vi "printgraph_V0.01.vi"(4 "AFR":refnum<vi>, 6 "AFR-Graph (Eingang)":refnum<vi>, 8 "Überschrift":refnum<vi>, 9 "Ergebnis":refnum<vi>, 10 "Fahrzeugdaten":refnum<vi>, 11 "PM-Graph (Eingang)":refnum<vi>) -> ()   [LabVIEW 2014]
uses:
  <vilib>/Utility/NIReport.llb/HTML Report Image Alignment.ctl
  <vilib>/Utility/NIReport.llb/Append Report Text (str wrap).vi
  <vilib>/Utility/NIReport.llb/NI_report.lvclass
  <vilib>/Utility/NIReport.llb/NI_ReportGenerationCore.lvlib
panel:
  out "AFR-Graph":cluster{dbl[], dbl[]}[](graph)
  out "PM-Graph":cluster{dbl[], dbl[]}[](graph)
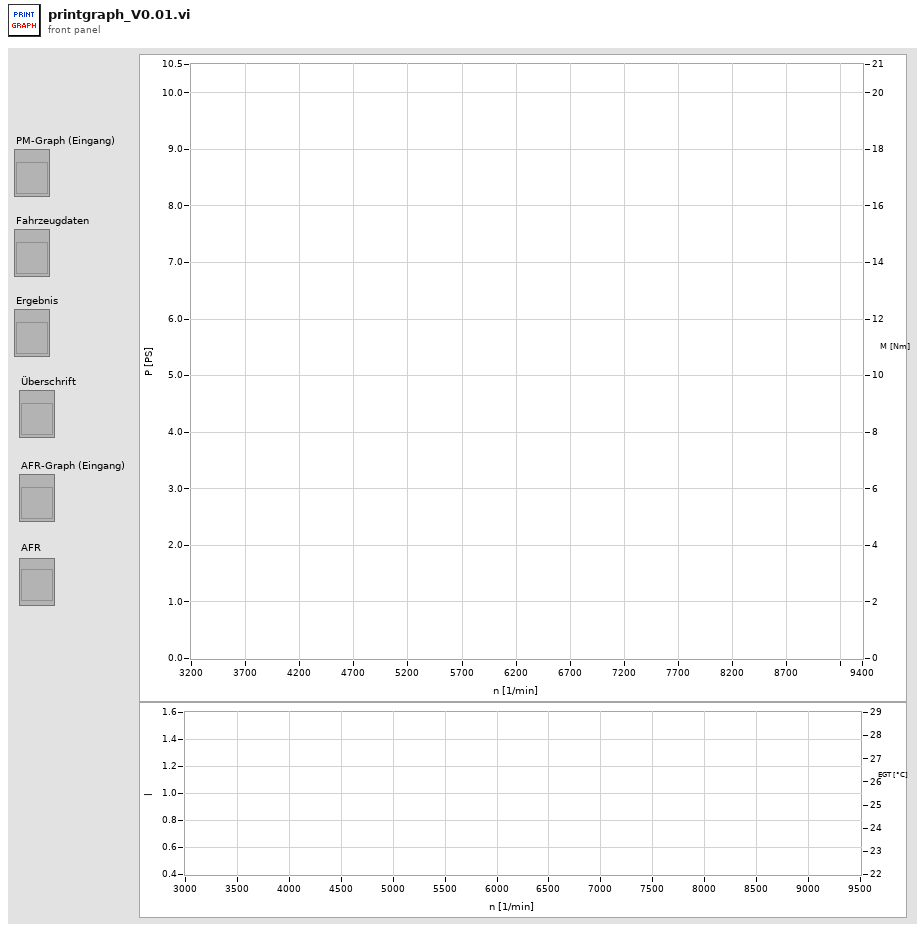
[diagram p1: front panel]
types:
  T1 = typedef "NI_ReportGenerationCore.lvlib/HTML Report Image Alignment.ctl" = enum16{"(default)", "LEFT", "RIGHT", "TOP", "TEXTTOP", "MIDDLE", "ABSMIDDLE", "BASELINE", "BOTTOM", "ABSBOTTOM"}
  T2 = cluster{"Charset (-1)":i16, "Weight (-1)":i16, "Name":string, "Size":string}
  T3 = cluster{"Italic":enum16{"Italic Unchanged", "Italic On", "Italic Off"}, "Strike Through":enum16{"Strike Through Unchanged", "Strike Through On", "Strike Through Off"}, "Underline":enum16{"Underline Unchanged", "Underline On", "Underline Off"}, "Bold":enum16{"Bold Unchanged", "Bold On", "Bold Off"}}
  T4 = typedef "LVRangeTypeDef.ctl" = cluster{"Minimum":dbl, "Maximum":dbl, "Increment":dbl, "Minor Increment":dbl, "Start":dbl}
  T5 = typedef "LVFontTypeDef.ctl" = cluster{"Font Name":string, "Size":u16, "Bold":bool, "Italic":bool, "Underline":bool, "Strikeout":bool, "Color":u32}
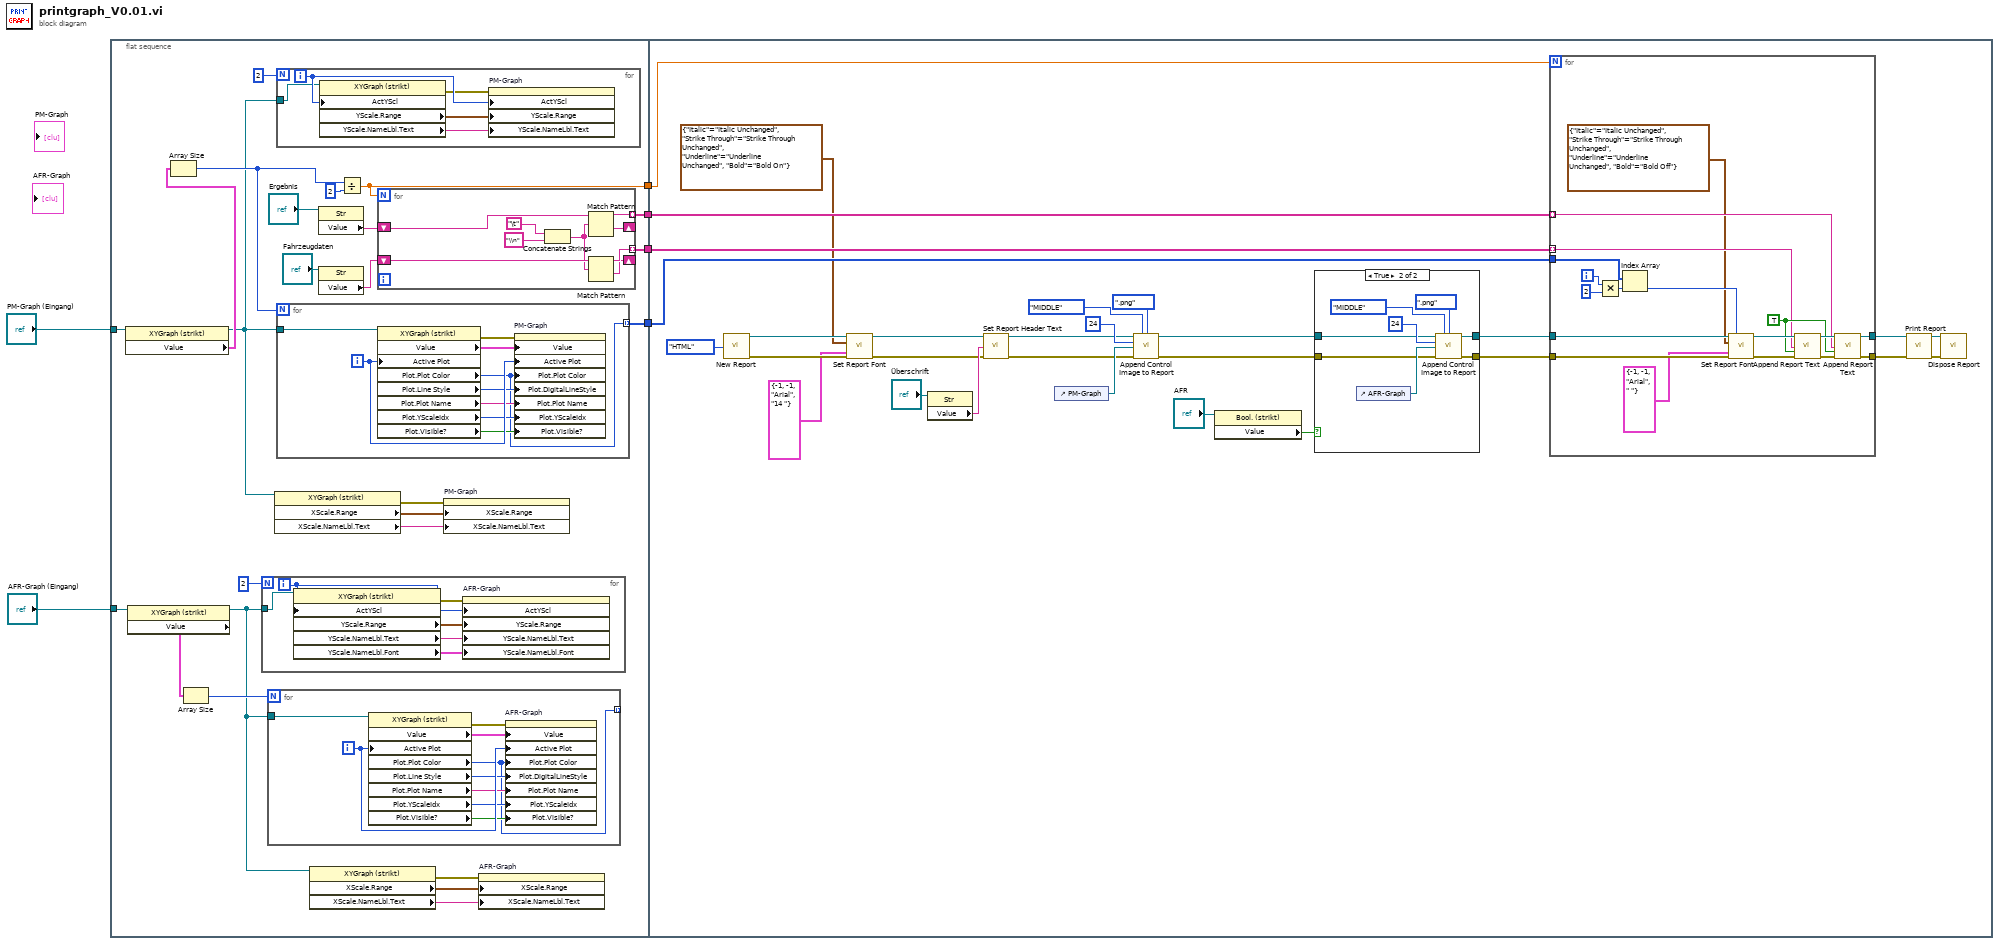
[diagram p0: block diagram]
diagram:
  n1 = flat-sequence {
    tunnel: "PM-Graph (Eingang)" -> [w31]
    tunnel: [w26] -> w5
    tunnel: [w23] -> w4
    tunnel: [w22] -> w3
    tunnel: [w20] -> w2
    tunnel: "AFR-Graph (Eingang)" -> [w13]
    tunnel: w5 -> [w90]
    tunnel: w4 -> [w89]
    tunnel: w3 -> [w88]
    tunnel: w2 -> [w87]
    frame #0 {
      n2 = property on="Eigenschaftsknoten" class="XYGraph (strikt)"(reference=w31) -> (reference out=w17:refnum<vi>, "Value"=w30:cluster{dbl[], dbl[]}[])  [unwired: 1 in, 1 out]
      n3 = property on="Eigenschaftsknoten" class="XYGraph (strikt)"(reference=w13) -> (reference out=w7:refnum<vi>, "Value"=w11:cluster{dbl[], dbl[]}[])  [unwired: 1 in, 1 out]
      n4 = Array Size(array=w30) -> (size(s)=w19:i32)
      n5 = Array Size(array=w11) -> (size(s)=w12:i32)
      n6 = for {
        N: 2 -> [_]
        tunnel: w7 -> [w44]
        i -> [w45]
        n7 = property on="Eigenschaftsknoten" class="XYGraph (strikt)"(reference=w44, "ActYScl"=w45) -> (error out=w42:errorcluster, "YScale.Range"=w46:T4, "YScale.NameLbl.Text"=w43:string, "YScale.NameLbl.Font"=w41:T5)  [unwired: 1 in, 1 out]
        n8 = property on="AFR-Graph" class="XYGraph (strikt)"(error in=w42, "ActYScl"=w45, "YScale.Range"=w46, "YScale.NameLbl.Text"=w43, "YScale.NameLbl.Font"=w41) -> ()  [unwired: 1 in, 2 out]
      }
      n9 = for {
        N: w12 -> [_]
        tunnel: w7 -> [w36]
        tunnel: [w32] -> _ mode=indexing
        i -> [w40]
        n10 = property on="Eigenschaftsknoten" class="XYGraph (strikt)"(reference=w36, "Active Plot"=w40) -> (error out=w33:errorcluster, "Value"=w34:cluster{dbl[], dbl[]}[], "Plot.Plot Color"=w32:u32, "Plot.Line Style"=w39:u8, "Plot.Plot Name"=w38:string, "Plot.YScaleIdx"=w37:u32, "Plot.Visible?"=w35:bool)  [unwired: 1 in, 1 out]
        n11 = property on="AFR-Graph" class="XYGraph (strikt)"(error in=w33, "Value"=w34, "Active Plot"=w40, "Plot.Plot Color"=w32, "Plot.DigitalLineStyle"=w39, "Plot.Plot Name"=w38, "Plot.YScaleIdx"=w37, "Plot.Visible?"=w35) -> ()  [unwired: 1 in, 2 out]
      }
      n12 = property on="Eigenschaftsknoten" class="XYGraph (strikt)"(reference=w17) -> (error out=w16:errorcluster, "XScale.Range"=w18:T4, "XScale.NameLbl.Text"=w15:string)  [unwired: 1 in, 1 out]
      n13 = for {
        N: 2 -> [_]
        tunnel: w17 -> [w58]
        i -> [w59]
        n14 = property on="Eigenschaftsknoten" class="XYGraph (strikt)"(reference=w58, "ActYScl"=w59) -> (error out=w56:errorcluster, "YScale.Range"=w60:T4, "YScale.NameLbl.Text"=w57:string)  [unwired: 1 in, 1 out]
        n15 = property on="PM-Graph" class="XYGraph (strikt)"(error in=w56, "ActYScl"=w59, "YScale.Range"=w60, "YScale.NameLbl.Text"=w57) -> ()  [unwired: 1 in, 2 out]
      }
      n16 = for {
        N: w19 -> [_]
        tunnel: w17 -> [w65]
        tunnel: [w61] -> w26 mode=indexing
        i -> [w69]
        n17 = property on="Eigenschaftsknoten" class="XYGraph (strikt)"(reference=w65, "Active Plot"=w69) -> (error out=w62:errorcluster, "Value"=w63:cluster{dbl[], dbl[]}[], "Plot.Plot Color"=w61:u32, "Plot.Line Style"=w68:u8, "Plot.Plot Name"=w67:string, "Plot.YScaleIdx"=w66:u32, "Plot.Visible?"=w64:bool)  [unwired: 1 in, 1 out]
        n18 = property on="PM-Graph" class="XYGraph (strikt)"(error in=w62, "Value"=w63, "Active Plot"=w69, "Plot.Plot Color"=w61, "Plot.DigitalLineStyle"=w68, "Plot.Plot Name"=w67, "Plot.YScaleIdx"=w66, "Plot.Visible?"=w64) -> ()  [unwired: 1 in, 2 out]
      }
      n19 = property on="Eigenschaftsknoten" class="XYGraph (strikt)"(reference=w7) -> (error out=w9:errorcluster, "XScale.Range"=w8:T4, "XScale.NameLbl.Text"=w10:string)  [unwired: 1 in, 1 out]
      n20 = property class="Str"(reference="Ergebnis") -> ("Value"=w25:string)  [unwired: 1 in, 2 out]
      n21 = property class="Str"(reference="Fahrzeugdaten") -> ("Value"=w24:string)  [unwired: 1 in, 2 out]
      n22 = Divide(x=w19, y=u32 2) -> (x/y=w20:dbl)
      n23 = for {
        N: w20 -> [_]
        tunnel: [w52] -> w23 mode=indexing
        tunnel: [w53] -> w22 mode=indexing
        shift-right: [w49] -> _
        shift-left: w25 -> [w55]
        shift-right: [w48] -> _
        shift-left: w24 -> [w54]
        n24 = Concatenate Strings("\t", "\\n" ("Regulärer Ausdruck")) -> (w51:string)
        n25 = Match Pattern(string=w55, regular expression=w51) -> (before substring=w52:string, after substring=w49:string)  [unwired: 1 in, 2 out]
        n26 = Match Pattern(string=w54, regular expression=w51) -> (before substring=w53:string, after substring=w48:string)  [unwired: 1 in, 2 out]
      }
      n27 = property on="PM-Graph" class="XYGraph (strikt)"(error in=w16, "XScale.Range"=w18, "XScale.NameLbl.Text"=w15) -> ()  [unwired: 1 in, 2 out]
      n28 = property on="AFR-Graph" class="XYGraph (strikt)"(error in=w9, "XScale.Range"=w8, "XScale.NameLbl.Text"=w10) -> ()  [unwired: 1 in, 2 out]
    }
    frame #1 {
      n29 = call <vilib>:"New Report.vi"("report type"=enum16{"Standard Report", "HTML"}."HTML") -> ("report out"=w82:refnum<class "NI_report.lvclass">, "error out"=w81:errorcluster)  [unwired: 13 in]
      n30 = call-dynamic "Set Report Font.vi"("report in"=w82, "text options"=T3 {"Italic"=enum."Italic Unchanged", "Strike Through"=enum."Strike Through Unchanged", "Underline"=enum."Underline Unchanged", "Bold"=enum."Bold On"}, "font settings"=T2 {"Charset (-1)"=-1, "Weight (-1)"=-1, "Name"="Arial", "Size"="14 "}, "error in (no error)"=w81) -> ("report out"=w79:refnum<class "NI_report.lvclass">, "error out"=w80:errorcluster)  [unwired: 9 in, 1 out]
      n31 = property on="Eigenschaftsknoten" class="Str"(reference="Überschrift") -> ("Value"=w83:string)  [unwired: 1 in, 2 out]
      n32 = call-dynamic "Set Report Header Text.vi"("report in"=w79, "center header text"=w83, "error in (no error)"=w80) -> ("report out"=w85:refnum<class "NI_report.lvclass">, "error out"=w86:errorcluster)  [unwired: 11 in]
      n33 = control-ref of="PM-Graph"() -> (w93:refnum<vi>)
      n34 = call-dynamic "Append Control Image to Report.vi"("report in"=w85, "alignment (default)"=HTML_Report_Image_Alignment."MIDDLE", "image file type (.jpg)"=enum16{".jpg", ".png"}.".png", "image depth"=24, "ctrl reference"=w93, "error in (no error)"=w86) -> ("report out"=w75:refnum<class "NI_report.lvclass">, "error out"=w74:errorcluster)  [unwired: 6 in, 2 out]
      n35 = property class="Bool. (strikt)"(reference="AFR") -> ("Value"=w70:bool)  [unwired: 1 in, 2 out]
      n36 = case shown="True" w70 {
        tunnel: w75 -> [w99 w104]
        tunnel: w74 -> [w100 w103]
        tunnel: [w100 w102] -> w73
        tunnel: [w99 w101] -> w72
        frame False {
        }
        frame True {
          n37 = control-ref of="AFR-Graph"() -> (w107:refnum<vi>)
          n38 = call-dynamic "Append Control Image to Report.vi"("report in"=w104, "alignment (default)"=HTML_Report_Image_Alignment."MIDDLE", "image file type (.jpg)"=enum16{".jpg", ".png"}.".png", "image depth"=24, "ctrl reference"=w107, "error in (no error)"=w103) -> ("report out"=w101:refnum<class "NI_report.lvclass">, "error out"=w102:errorcluster)  [unwired: 6 in, 2 out]
        }
      }
      n39 = for {
        N: w87 -> [_]
        tunnel: w73 -> [w124]
        tunnel: [w119] -> w91
        tunnel: w72 -> [w126]
        tunnel: [w120] -> w92
        tunnel: w90 -> [w117]
        tunnel: w89 -> [w112] mode=indexing
        tunnel: w88 -> [w111] mode=indexing
        i -> [w115]
        w118 = TRUE
        n40 = Multiply(x=w115, y=2) -> (x*y=w116:i32)
        n41 = Index Array(array=w117, index=w116) -> (element=w113:u32)
        n42 = call-dynamic "Set Report Font.vi"("report in"=w126, "text color (unchanged)"=w113, "text options"=T3 {"Italic"=enum."Italic Unchanged", "Strike Through"=enum."Strike Through Unchanged", "Underline"=enum."Underline Unchanged", "Bold"=enum."Bold Off"}, "font settings"=T2 {"Charset (-1)"=-1, "Weight (-1)"=-1, "Name"="Arial", "Size"=" "}, "error in (no error)"=w124) -> ("report out"=w125:refnum<class "NI_report.lvclass">, "error out"=w123:errorcluster)  [unwired: 8 in, 1 out]
        n43 = call-poly <vilib>:"Append Report Text.vi"("report in"=w125, "text"=w111, "append on new line? (F)"=w118, "error in (no error)"=w123) -> ("report out"=w122:refnum<class "NI_report.lvclass">, "error out"=w121:errorcluster)  [unwired: 8 in, 2 out]
        n44 = call-poly <vilib>:"Append Report Text.vi"("report in"=w122, "text"=w112, "append on new line? (F)"=w118, "error in (no error)"=w121) -> ("report out"=w120:refnum<class "NI_report.lvclass">, "error out"=w119:errorcluster)  [unwired: 8 in, 2 out]
      }
      n45 = call-dynamic "Print Report.vi"("report in"=w92, "error in (no error)"=w91) -> ("report out"=w97:refnum<class "NI_report.lvclass">, "error out"=w98:errorcluster)  [unwired: 12 in]
      n46 = call-dynamic "Dispose Report.vi"("report in"=w97, "error in (no error)"=w98) -> ()  [unwired: 13 in, 1 out]
    }
  }
